vi "Delete same Elements from 1D Array (String)__ogtk.vi"(11 "array in":string[](array[string])) -> (3 "array out":string[](array[string]))   [LabVIEW 2017]
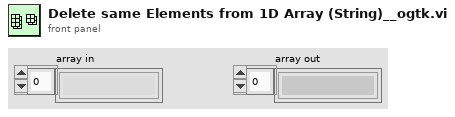
[diagram p1: front panel]
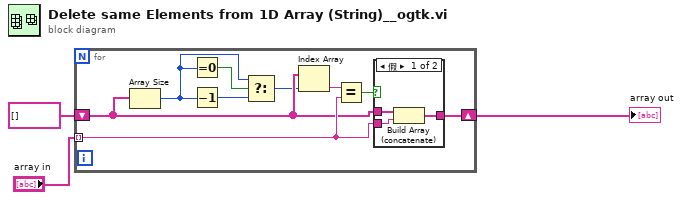
[diagram p0: block diagram]
diagram:
  n1 = for {
    shift-right: [w11] -> w1
    shift-left: string[] [] -> [w10]
    tunnel: "array in" -> [w12] mode=indexing
    n2 = Array Size(array=w10) -> (size(s)=w4:i32)
    n3 = Equal To 0?(x=w4) -> (x = 0?=w7:bool)
    n4 = Decrement(x=w4) -> (x-1=w5:i32)
    n5 = Select(t=w4, s=w7, f=w5) -> (s? t:f=w6:i32)
    n6 = Index Array(array=w10, index=w6) -> (element=w8:string)
    n7 = Equal?(x=w8, y=w12) -> (x = y?=w9:bool)
    n8 = case shown="假" w9 {
      tunnel: w12 -> [w13 _]
      tunnel: [w15 w16] -> w11
      tunnel: w10 -> [w14 w16]
      frame False {
        n9 = Build Array (concatenate)(w14, w13) -> (w15:string[])
      }
      frame True {
      }
    }
  }
  "array out" <- w1
